vi "acq.saveLight.vi"(5 "vars":T2={"save"={"base_folder"={"Folder"=path "", "tif"=FALSE, "jpg"=FALSE}, "module"="", "#"=20, "sub#"=0, "save.op"=enum."Full", "same?"=FALSE, "Shift"=enum."Single", "jpg?"=FALSE, "flip"={"x"=FALSE, "y"=FALSE}}, "acq"={"# Acq"=100}, "calib.manual"={"BG"={"Image"=[], "enabled?"=FALSE}, "FF"={"Image"=[], "enabled?"=FALSE}}}, 7 "path":T1, 8 "error in":errorcluster, 9 "Dark":u16[][](array[numeric]), 10 "PL":u16[][](array[numeric]), 11 "Bright":u16[][](array[numeric])) -> (0 "error out":errorcluster, 2 "PL":u16[][](array[numeric]), 3 "IR":u16[][](array[numeric]))   [LabVIEW 2020]
uses:
  _controls/data.vars.ctl
  _controls/flip.ctl
  _controls/path.ctl
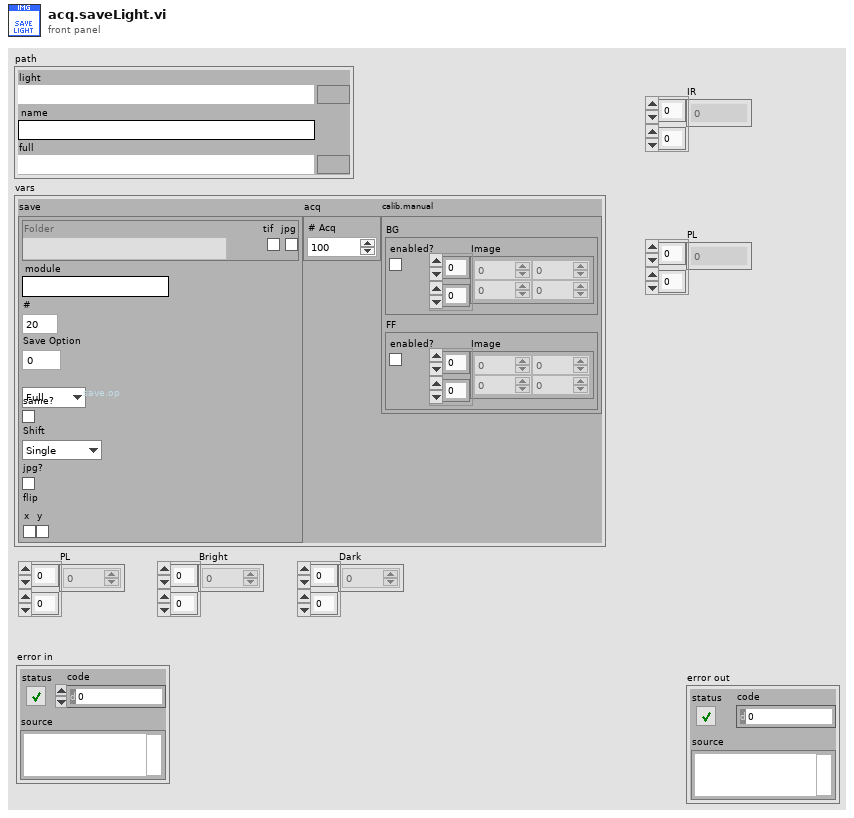
[diagram p1: front panel]
types:
  T1 = typedef "path.ctl" = cluster{"light":path, "name":string, "full":path}
  T2 = typedef "data.vars.ctl" = cluster{"save":cluster{"base_folder":cluster{"Folder":path, "tif":bool, "jpg":bool}, "module":string, "#":u32, "sub#":u8, "save.op":enum16{"Full", "Light"}, "same?":bool, "Shift":enum16{"Single", "Leapfrog"}, "jpg?":bool, "flip":T3}, "acq":cluster{"# Acq":u16}, "calib.manual":cluster{"BG":cluster{"Image":u16[][], "enabled?":bool}, "FF":cluster{"Image":u16[][], "enabled?":bool}}}
  T3 = typedef "flip.ctl" = cluster{"x":bool, "y":bool}
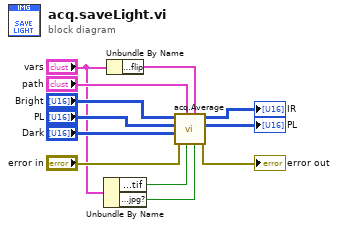
[diagram p0: block diagram]
diagram:
  n1 = Unbundle By Name("vars") -> ("save.base_folder.tif"=w4:bool, "save.jpg?"=w3:bool)
  n2 = Unbundle By Name("vars") -> ("save.flip"=w1:T3)
  n3 = call "acq.Average.vi"("jpg?"=w3, "flip"=w1, "Save"=w4, "path"="path", "error in"="error in", "Dark"="Dark", "PL"="PL", "Bright"="Bright") -> ("error out"=→"error out":errorcluster, "PL"=→"PL":u16[][], "IL"=→"IR":u16[][])  [unwired: 1 in]
